vi "configureHWIO_1_exposureTrigger.vi"(8 "error in (no error)":errorcluster, 9 "polarity":u16(ring)=4 items=["rising edge"=4, "falling edge"=8], 10 "on":bool=TRUE, 11 "Camera in":refnum<class "Camera.lvclass">) -> (0 "error out":errorcluster, 3 "Camera out":refnum<class "Camera.lvclass">)   [LabVIEW 2019, in "Camera.lvclass"]
doc: "Configures HWIO exposure trigger for polarity and status (enabled / disabled). Generates an error if camera is recording or if HWIO configuration is not supported."
uses:
  Camera.lvclass
  pco.sdk/CameraDescription/CameraDescription.lvlib
  pco.sdk/TimingControl/TimingControl.lvlib
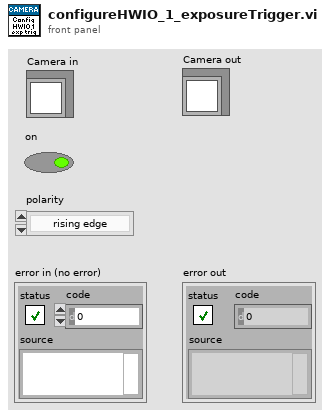
[diagram p1: front panel]
types:
  T1 = cluster{"wSensorTypeDESC":u16, "wSensorSubTypeDESC":u16, "wMaxHorzResStdDESC":u16, "wMaxVertResStdDESC":u16, "wMaxHorzResExtDESC":u16, "wMaxVertResExtDESC":u16, "wDynResDESC":u16, "wMaxBinHorzDESC":u16, "wBinHorzSteppingDESC":u16, "wMaxBinVertDESC":u16, "wBinVertSteppingDESC":u16, "wRoiHorStepsDESC":u16, "wRoiVertStepsDESC":u16, "wNumADCsDESC":u16, "wMinSizeHorzDESC":u16, "dwPixelRateDESC":u32[], "wConvFactDESC":u16[], "sCoolingSetpoints":i16[], "wSoftRoiHorStepsDESC":u16, "wSoftRoiVertStepsDESC":u16, "wIRDESC":u16, "wMinSizeVertDESC":u16, "dwMinDelayDESC":u32, "dwMaxDelayDESC":u32, "dwMinDelayStepDESC":u32, "dwMinExposureDESC":u32, "dwMaxExposureDESC":u32, "dwMinExposureStepDESC":u32, "dwMinDelayIRDESC":u32, "dwMaxDelayIRDESC":u32, "dwMinExposureIRDESC":u32, "dwMaxExposureIRDESC":u32, "wTimeTableDESC":u16, "wDoubleImageDESC":u16, "sMinCoolSetDESC":i16, "sMaxCoolSetDESC":i16, "sDefaultCoolSetDESC":i16, "wPowerDownModeDESC":u16, "wOffsetRegulationDESC":u16, "wColorPatternDESC":u16, "wPatternTypeDESC":u16, "wNumCoolingSetpoints":u16, "dwGeneralCapsDESC1":u32, "dwGeneralCapsDESC2":u32, "dwExtSyncFrequency":u32[], "dwGeneralCapsDESC3":u32, "dwGeneralCapsDESC4":u32}
  T2 = cluster{"wSignalNum":u16, "wEnabled":u16, "wType":u16, "wPolarity":u16, "wFilterSetting":u16, "wSelected":u16, "dwParameter":u32[], "dwSignalFunctionality":u32[]}
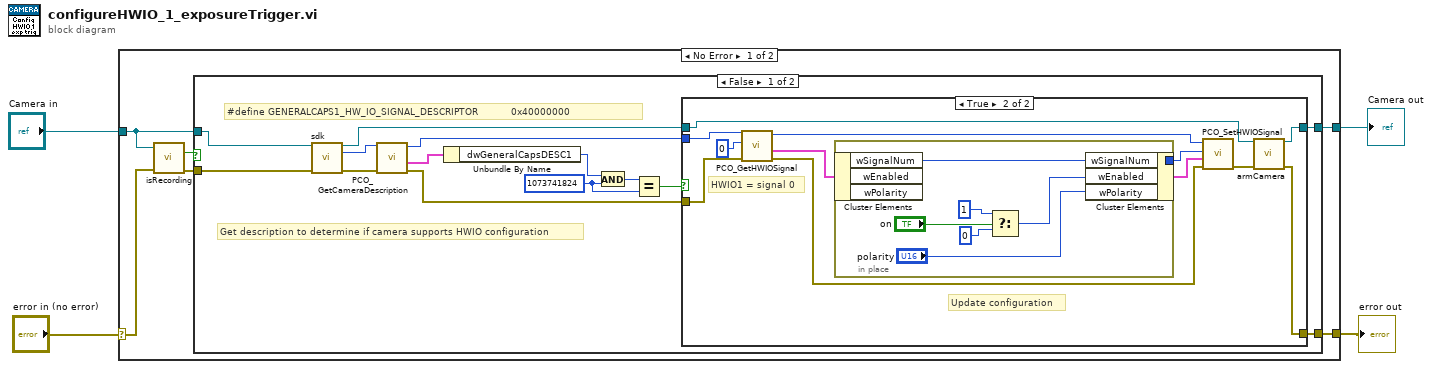
[diagram p0: block diagram]
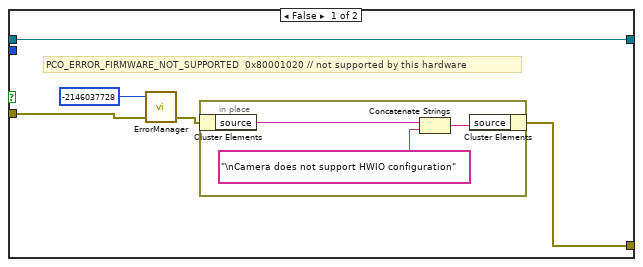
[diagram p2: hidden frame]
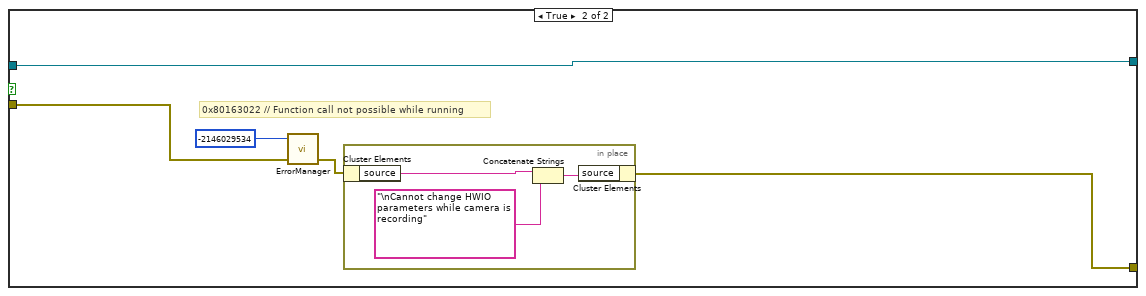
[diagram p3: hidden frame]
diagram:
  n1 = case shown="No Error" "error in (no error)" {
    selector: "error in (no error)" -> [w6 w60]
    tunnel: [w8 w60] -> w3
    tunnel: "Camera in" -> [w10 w59]
    tunnel: [w7 w59] -> w1
    frame No Error {
      n2 = call-dynamic "isRecording.vi"("Camera in"=w10, "error in (no error)"=w6) -> ("recording"=w9:bool, "error out"=w5:errorcluster)  [unwired: 11 in, 1 out]
      n3 = case shown="False" w9 {
        tunnel: w10 -> [w24 w51]
        tunnel: w5 -> [w12 w54]
        tunnel: [w15 w52] -> w8
        tunnel: [w14 w51] -> w7
        frame False {
          w19 = u32 1073741824 ("y")
          # "Get description to determine if camera supports HWIO configuration"
          # "#define GENERALCAPS1_HW_IO_SIGNAL_DESCRIPTOR           0x40000000"
          n4 = call-dynamic "sdk.vi"("Camera in"=w24, "error in (no error)"=w12) -> ("Camera out"=w16:refnum<class "Camera.lvclass">, "sdk"=w23:u64, "error out"=w13:errorcluster)  [unwired: 11 in]
          n5 = call "PCO_GetCameraDescription.vi"("error in (no error)"=w13, "ph"=w23) -> ("error out"=w11:errorcluster, "strDescription"=w22:T1, "ph out"=w17:u64)  [unwired: 6 in, 1 out]
          n6 = Unbundle By Name(w22) -> ("dwGeneralCapsDESC1"=w21:u32)
          n7 = And(x=w21, y=w19) -> (x .and. y?=w20:u32)
          n8 = Equal?(x=w20, y=w19) -> (x = y?=w18:bool)
          n9 = case shown="True" w18 {
            tunnel: w11 -> [w29 w42]
            tunnel: [w26 w36] -> w15
            tunnel: w17 -> [_ w44]
            tunnel: w16 -> [w25 w34]
            tunnel: [w25 w33] -> w14
            frame False {
              # "PCO_ERROR_FIRMWARE_NOT_SUPPORTED  0x80001020 // not supported by this hardware"
              n10 = call "ErrorManager.vi"("error in (no error)"=w29, "error code"=-2146037728) -> ("error out"=w27:errorcluster)  [unwired: 2 in, 1 out]
              n11 = in-place {
                n12 = in-place-cluster #1(w27) -> ("source"=w32:string)
                n13 = Concatenate Strings(w32, "\nCamera does not support HWIO configuration") -> (w30:string)
                n14 = in-place-cluster #1("source"=w30) -> (w26:errorcluster)
              }
            }
            frame True {
              # "Update configuration"
              # "HWIO1 = signal 0"
              n15 = call "PCO_GetHWIOSignal.vi"("error in (no error)"=w42, "wSignalNum"=u16 0, "ph"=w44) -> ("error out"=w35:errorcluster, "strSignal"=w41:T2, "ph out"=w40:u64)  [unwired: 5 in, 1 out]
              n16 = in-place {
                in-place-border: [w45] -> w39
                n17 = in-place-cluster #2(w41) -> ("wSignalNum"=w45:u16)  [unwired: 2 out]
                n18 = Select(t=u16 1 ("wEnabled"), s="on", f=u16 0 ("wEnabled")) -> (s? t:f=w48:u16)
                n19 = in-place-cluster #2("wSignalNum"=w45, "wEnabled"=w48, "wPolarity"="polarity") -> (w38:T2)
              }
              n20 = call "PCO_SetHWIOSignal.vi"("error in (no error)"=w35, "strSignal"=w38, "wSignalNum"=w39, "ph"=w40) -> ("error out"=w37:errorcluster)  [unwired: 5 in, 2 out]
              n21 = call-dynamic "armCamera.vi"("Camera in"=w34, "error in (no error)"=w37) -> ("Camera out"=w33:refnum<class "Camera.lvclass">, "error out"=w36:errorcluster)  [unwired: 12 in]
            }
          }
        }
        frame True {
          # "0x80163022 // Function call not possible while running"
          n22 = call "ErrorManager.vi"("error in (no error)"=w54, "error code"=-2146029534) -> ("error out"=w53:errorcluster)  [unwired: 2 in, 1 out]
          n23 = in-place {
            n24 = in-place-cluster #3(w53) -> ("source"=w58:string)
            n25 = Concatenate Strings(w58, "\nCannot change HWIO parameters while camera is recording") -> (w56:string)
            n26 = in-place-cluster #3("source"=w56) -> (w52:errorcluster)
          }
        }
      }
    }
    frame Error {
    }
  }
  "Camera out" <- w1
  "error out" <- w3
